vi "Save Profile.vi"(9 "Profile":string[][](array[string]), 10 "Current Profile":string, 11 "Profiles Path":path) -> (3 "Profile OUT":string[][](array[string]))   [LabVIEW 2019]
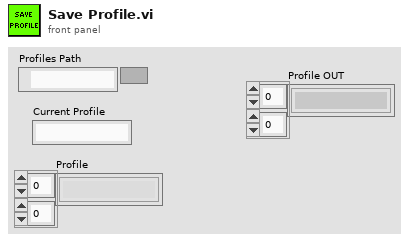
[diagram p1: front panel]
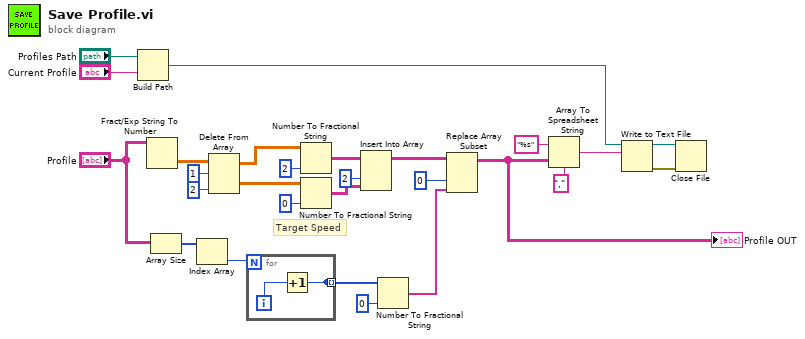
[diagram p0: block diagram]
diagram:
  # "Target Speed"
  n1 = Build Path(base path="Profiles Path", name or relative path="Current Profile") -> (appended path=w27:path)
  n2 = Fract/Exp String To Number(string="Profile") -> (number=w10:dbl[][])  [unwired: 3 in, 1 out]
  n3 = Array Size(array="Profile") -> (size(s)=w20:i32[])
  n4 = Index Array(array=w20) -> (element=w19:i32)  [unwired: 1 in]
  n5 = Delete From Array(array=w10, length=1, index (col)=2 ("disabled index (col)")) -> (deleted portion=w6:dbl[][], array with subset deleted=w5:dbl[][])  [unwired: 1 in]
  n6 = for {
    N: w19 -> [_]
    tunnel: [w28] -> _ mode=indexing
    tunnel: [w28] -> w18 mode=indexing
    i -> [w29]
    n7 = Increment(x=w29) -> (x+1=w28:i32)
  }
  n8 = Number To Fractional String(number=w5, precision (6)=i16 2) -> (F-format string=w4:string[][])  [unwired: 2 in]
  n9 = Number To Fractional String(number=w6, precision (6)=i16 0) -> (F-format string=w3:string[][])  [unwired: 2 in]
  n10 = Insert Into Array(array=w4, index (col)=2 ("disabled index (col)"), new element=w3) -> (w1:string[][])  [unwired: 1 in]
  n11 = Number To Fractional String(number=w18, precision (6)=i16 0) -> (F-format string=w16:string[])  [unwired: 2 in]
  n12 = Replace Array Subset(array=w1, new element=w16, index (col)=0 ("disabled index (col)")) -> (w13:string[][])  [unwired: 1 in]
  "Profile OUT" <- w13
  n13 = Array To Spreadsheet String(delimiter (Tab)=",", array=w13, 3:"%s" ("format string")) -> (spreadsheet string=w14:string)
  n14 = Write to Text File(file (use dialog)=w27, text=w14) -> (refnum out=w26:refnum<file>, error out=w25:errorcluster)  [unwired: 2 in, 1 out]
  n15 = Close File(refnum=w26, error in=w25) -> ()  [unwired: 2 out]
